vi "Simple Example (with Encryption).vi"() -> ()   [LabVIEW 2019]
doc: "This example shows a simple encryption of log arguments. Encrypted arguments are implemented with bracketed key-value wildcard pairs. The wildcard is specified by:\n\n{wildcard} in the event data string; and arguments are single or lists of strings. \n\nThis shows how the console will encrypt data on the output and how it is decrypted on the read side."
uses:
  Log/Event Level.ctl
  Encryption/FFT/FFT.lvclass
  C:/Development/Open Source/tsc-event-logger/Encryption/Encryption.lvclass
  Log/Log.lvclass/Log.ctl
  Layouts/JSONLayout/JSONLayout.lvclass
  C:/Development/Open Source/tsc-event-logger/Layouts/Layout.lvclass
  cd0cdadd-5bba-4876-b4a7-6d6dc25bebc9.vi
  0255d82c-ae35-4f1c-bf70-cf29c14a7855.vi
  d915b4c3-683c-4e5b-a72c-46a47fdfc3fe.vi
  Log/Read Sinks.vi
  Log Sinks/Sink-Console/Sink-Console.lvclass
  C:/Development/Open Source/tsc-event-logger/Log Sinks/Log Sinks.lvclass
  Log Sinks/Sink-Console/Construct - Input.vi
  Log Sinks/Send Log Packet.vi
  Log/Log.lvclass
  TSC Event Logger.lvlib
  Encryption/Encryption.lvclass
panel:
  out "Decrypted messages":string
  in  "Record Event with multiple arg":bool
  in  "Record Event with arg":bool
  in  "Argument List":string[](array[string])
  in  "Single Argument":string
  in  "Add JSON Console":bool
  out "Second Console":string
  out "String":string
  in  "Level":T1=enum."INFO"
  in  "Record Event":bool
  in  "Event Data":string="test"
  out "Error Out":errorcluster
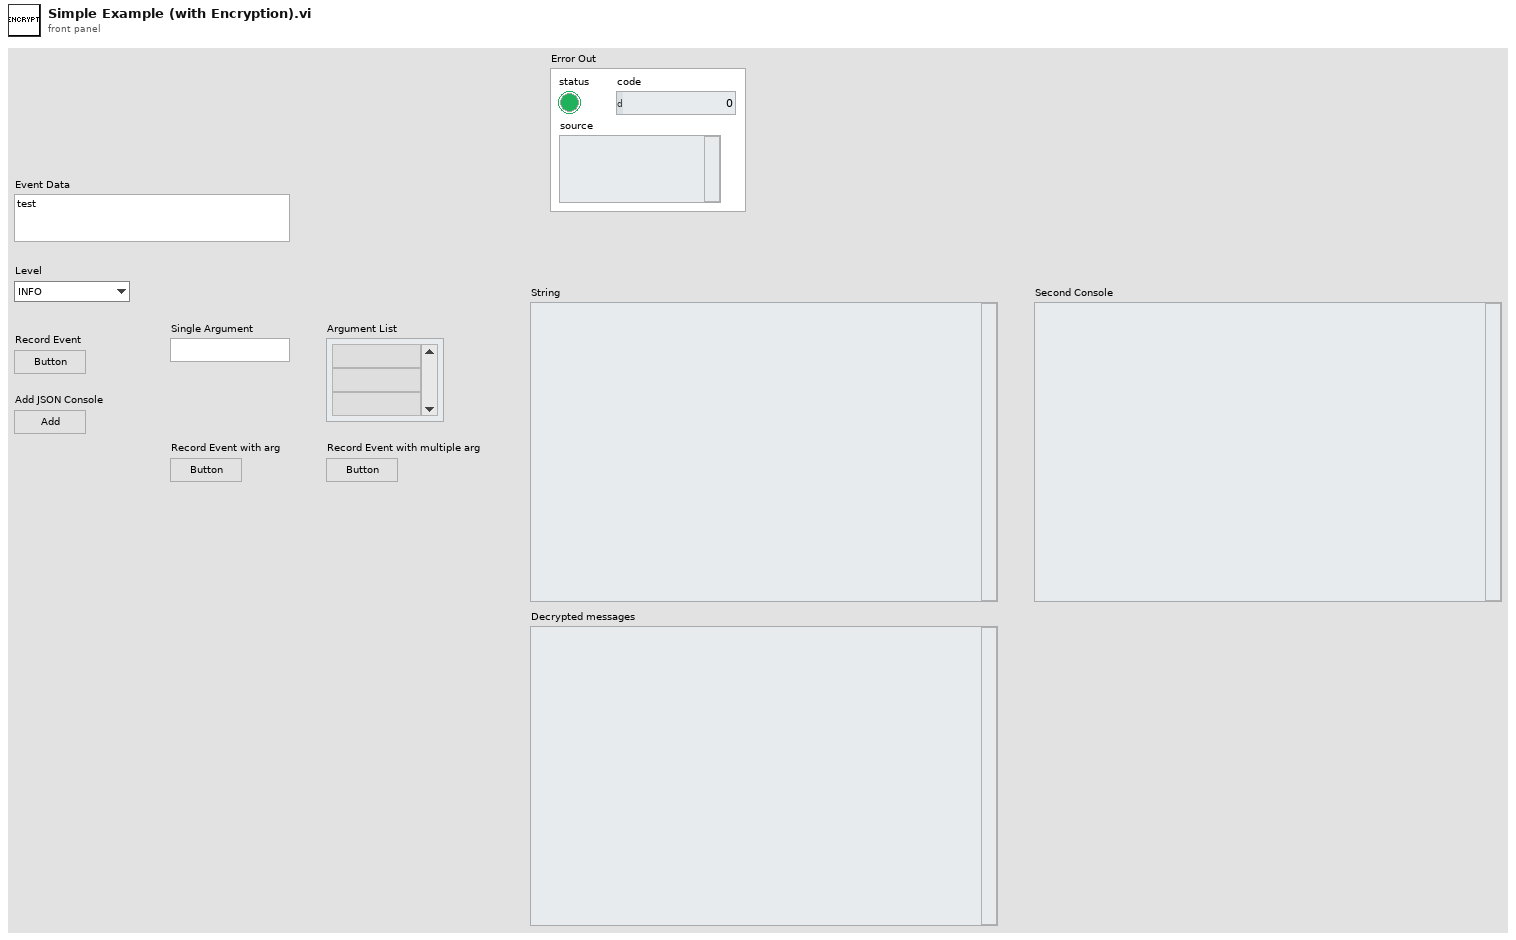
[diagram p1: front panel]
types:
  T1 = typedef "TSC Event Logger.lvlib/Event Level.ctl" = enum16{"OFF", "TRACE", "DEBUG", "INFO", "WARN", "ERROR", "FATAL"}
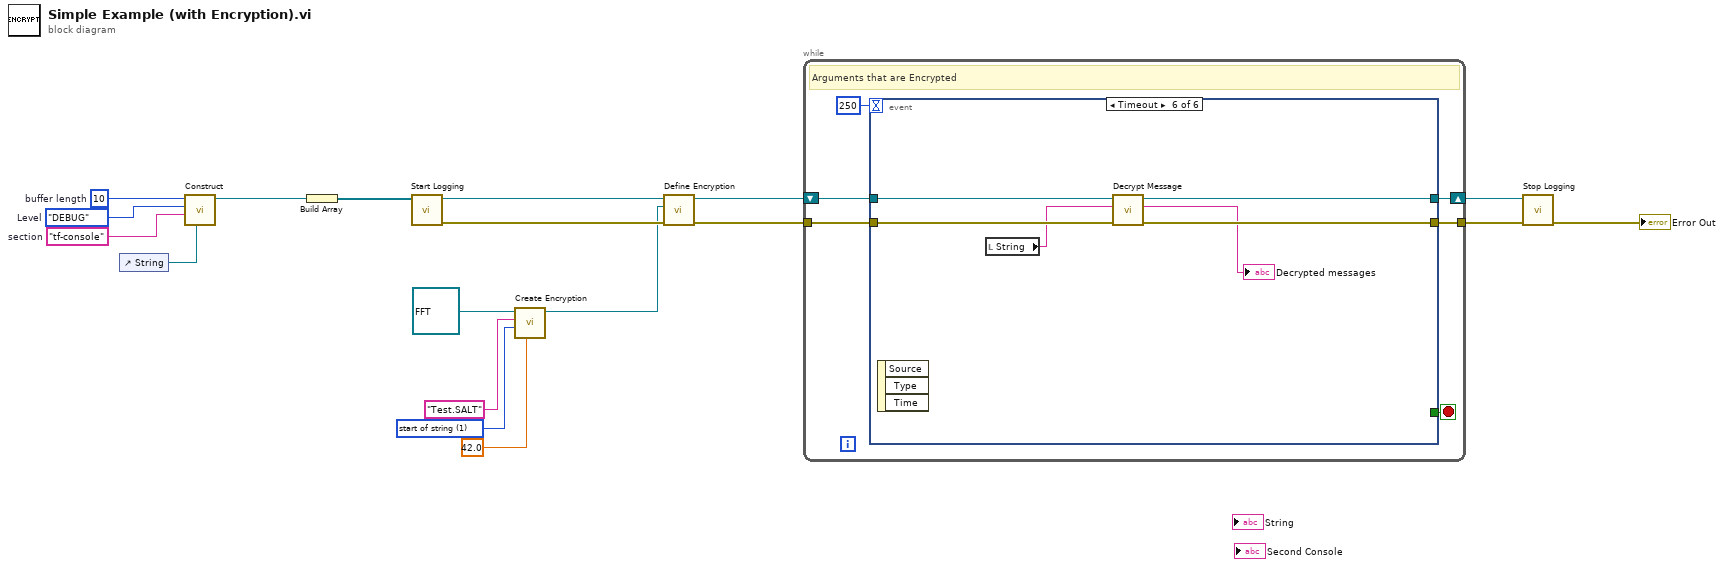
[diagram p0: block diagram]
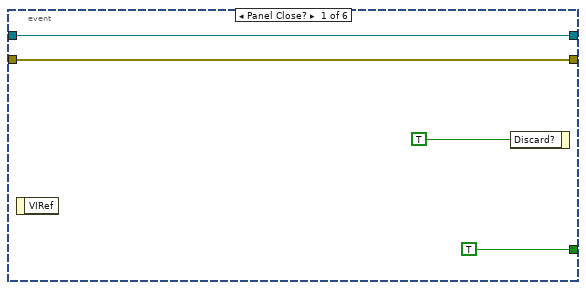
[diagram p2: hidden frame]
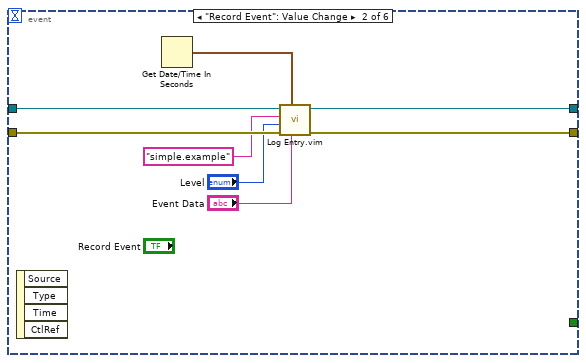
[diagram p3: hidden frame]
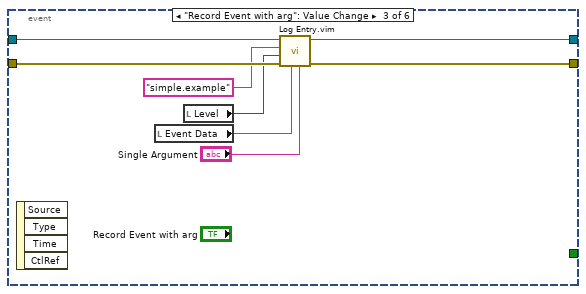
[diagram p4: hidden frame]
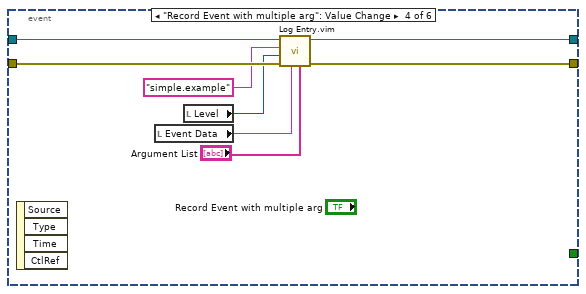
[diagram p5: hidden frame]
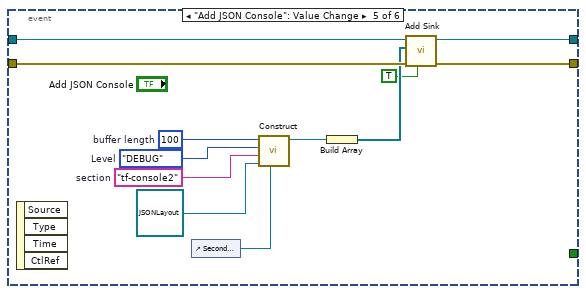
[diagram p6: hidden frame]
diagram:
  w6 = u16 1 items=["both", "start of string", "end of string"] ("SALT location (start of string)")
  w10 = 10  # buffer length
  w11 = Event_Level."DEBUG"  # Level
  w12 = "tf-console"  # section
  n1 = control-ref of="String"() -> (w13:refnum<vi>)
  n2 = call-poly "Construct.vi"("Console Ref"=w13, "Name"=w12, "Level"=w11, "buffer length"=w10) -> ("Sink-Console"=w14:refnum<class "Sink-Console.lvclass">)  [unwired: 6 in, 1 out]
  n3 = Build Array(w14) -> (w9:refnum<class "Sink-Console.lvclass">[])
  n4 = call "Start Logging.vi"("Sinks"=w9) -> ("Error Out"=w3:errorcluster, "Logger"=w15:refnum<class "Log.lvclass">)  [unwired: 9 in]
  n5 = call "Create Encryption.vi"("Multiplier"=42.0, "SALT location (start of string)"=w6, "SALT"="Test.SALT", "Encryption Method"=refnum<class "FFT.lvclass"> refnum ("TSC Event Logger.lvlib:FFT.lvclass")) -> ("Encryption output"=w2:refnum<class "FFT.lvclass">)  [unwired: 6 in, 1 out]
  n6 = call "Define Encryption.vi"("error in (no error)"=w3, "Encryption Method"=w2, "Log in"=w15) -> ("error out"=w1:errorcluster, "Log out"=w4:refnum<class "Log.lvclass">)  [unwired: 7 in]
  n7 = while {
    tunnel: w1 -> [w23]
    shift-right: [w21] -> w17
    shift-left: w4 -> [w22]
    tunnel: [w20] -> w16
    stop <- w24 stop-if-true
    # "Arguments that are Encrypted"
    n8 = event shown="[5] Timeout" {
      selector: _ -> [_ _ _ _ _ _]
      dyn-events: _ -> [_ _ _ _ _ _]
      timeout: 250 -> [_ _ _ _ _ _]
      tunnel: [TRUE _ _ _ _ _] -> w24
      tunnel: w23 -> [w25 w34 w42 w50 w64 w67]
      tunnel: w22 -> [w26 w36 w44 w52 w62 w70]
      tunnel: [w26 w35 w43 w51 w61 w69] -> w21
      tunnel: [w25 w33 w41 w49 w63 w68] -> w20
      event Panel Close? {
        n9 = event-data() -> ()  [unwired: 1 in, 1 out]
        n10 = event-data("Discard?"=TRUE) -> ()  [unwired: 1 in, 1 out]
      }
      event "Record Event": Value Change {
        n11 = event-data() -> ()  [unwired: 1 in, 4 out]
        n12 = Get Date/Time In Seconds() -> (seconds since 1Jan1904=w31:timestamp)
        n13 = call "Log Entry.vim"("Message"="Event Data", "Time"=w31, "error in (no error)"=w34, "Level"="Level", "Logger"="simple.example", "Log in"=w36) -> ("error out"=w33:errorcluster, "Log out"=w35:refnum<class "Log.lvclass">)  [unwired: 4 in]
      }
      event "Record Event with arg": Value Change {
        n14 = event-data() -> ()  [unwired: 1 in, 4 out]
        n15 = local read "Event Data"() -> (w38:string)
        n16 = local read "Level"() -> (w39:T1)
        n17 = call "Log Entry.vim"("Arguments"="Single Argument", "Message"=w38, "error in (no error)"=w42, "Level"=w39, "Logger"="simple.example", "Log in"=w44) -> ("error out"=w41:errorcluster, "Log out"=w43:refnum<class "Log.lvclass">)  [unwired: 4 in]
      }
      event "Record Event with multiple arg": Value Change {
        n18 = event-data() -> ()  [unwired: 1 in, 4 out]
        n19 = local read "Event Data"() -> (w46:string)
        n20 = local read "Level"() -> (w47:T1)
        n21 = call "Log Entry.vim"("Arguments"="Argument List", "Message"=w46, "error in (no error)"=w50, "Level"=w47, "Logger"="simple.example", "Log in"=w52) -> ("error out"=w49:errorcluster, "Log out"=w51:refnum<class "Log.lvclass">)  [unwired: 4 in]
      }
      event "Add JSON Console": Value Change {
        w60 = 100  # buffer length
        w59 = Event_Level."DEBUG"  # Level
        w58 = "tf-console2"  # section
        n22 = event-data() -> ()  [unwired: 1 in, 4 out]
        n23 = control-ref of="Second Console"() -> (w57:refnum<vi>)
        n24 = call-poly "Construct.vi"("Console Ref"=w57, "Layout Type"=refnum<class "JSONLayout.lvclass"> refnum ("TSC Event Logger.lvlib:JSONLayout.lvclass"), "Name"=w58, "Level"=w59, "buffer length"=w60) -> ("Sink-Console"=w56:refnum<class "Sink-Console.lvclass">)  [unwired: 5 in, 1 out]
        n25 = Build Array(w56) -> (w55:refnum<class "Sink-Console.lvclass">[])
        n26 = call "Add Sink.vi"("Include Encryption"=TRUE, "Error In"=w64, "Sinks"=w55, "Logger in"=w62) -> ("Error Out"=w63:errorcluster, "Logger"=w61:refnum<class "Log.lvclass">)  [unwired: 6 in]
      }
      event Timeout {
        n27 = event-data() -> ()  [unwired: 1 in, 3 out]
        n28 = local read "String"() -> (w65:string)
        n29 = call "Decrypt Message.vi"("Error In"=w67, "Message"=w65, "Log in"=w70) -> ("Error Out"=w68:errorcluster, "Decrypted Message"=→"Decrypted messages":string, "Log out"=w69:refnum<class "Log.lvclass">)  [unwired: 6 in]
      }
    }
  }
  n30 = call "Stop Logging.vi"("Error In"=w16, "Logger"=w17) -> ("Error Out"=→"Error Out":errorcluster)  [unwired: 8 in, 1 out]
